vi "terminal.vi"   [LabVIEW 2016]
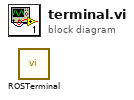
[diagram p0: block diagram]
diagram:
  n1 = call <userlib>:"ROSTerminal.vi"() -> ()  [unwired: 2 in]
